vi "Autonomous Independent.vi"() -> ()   [LabVIEW 2015]
doc: "This VI is called when autonomous begins, and will automatically be terminated when autonomous ends. You can carry out timed or sensor driven robot movement independently without needing to return to the caller."
uses:
  <vilib>/Rock Robotics/WPI/Solenoid/WPI_SolenoidValue.ctl
  <vilib>/Rock Robotics/WPI/Relay/WPI_RelayValue.ctl
  <vilib>/Rock Robotics/WPI/Utilities/WPI_GetSetVariantRefNum.vi
  <vilib>/Rock Robotics/Network Tables/NT Read String.vi
  <vilib>/Rock Robotics/WPI/RobotDrive/WPI_RobotDriveArcadeDrive_Standard(NoSaturation).vi
  <vilib>/Rock Robotics/Network Tables/NT Write Numeric Array.vi
  <vilib>/Rock Robotics/WPI/Solenoid/WPI_SolenoidSetEnum.vi
  Robot Global Data.vi
panel:
  out "Current Movement, for debugging":T1 {"Y Joystick Value" scale=1.0..-1.0; "X Joystick Value" scale=-1.0..1.0}
  in  "Array of robot movements":T2(array[cluster])=[{"X Joystick Value"=0.39393939393939403, "Y Joystick Value"=0.0, "Delay (sec)"=1.0, "Movement Name"="turn"}, {"X Joystick Value"=-0.3737373737373737, "Y Joystick Value"=0.0, "Delay (sec)"=1.0, "Movement Name"="turn back"}] {"Y Joystick Value" scale=1.0..-1.0; "X Joystick Value" scale=-1.0..1.0}
  # "Be sure to right-click and choose Data Operations>>Make Current Value default if you want to save the array values with the VI"
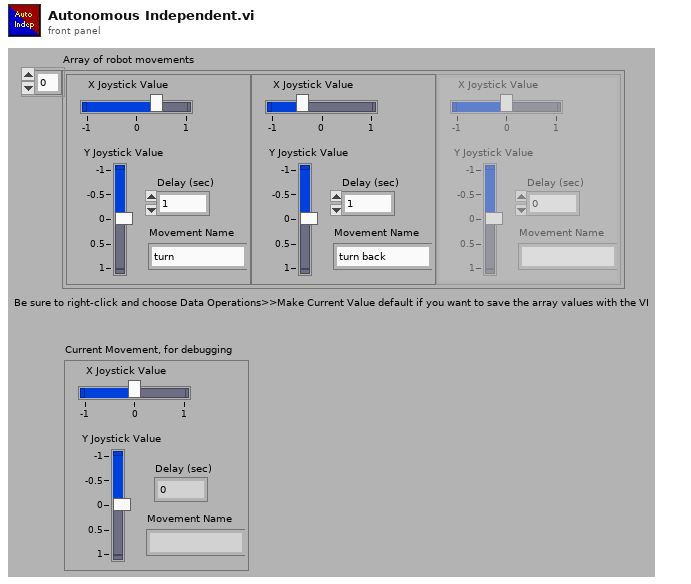
[diagram p1: front panel]
types:
  T1 = cluster{"X Joystick Value":dbl, "Y Joystick Value":dbl, "Delay (sec)":dbl, "Movement Name":string}
  T2 = cluster{"X Joystick Value":dbl, "Y Joystick Value":dbl, "Delay (sec)":dbl, "Movement Name":string}[]
  T3 = typedef "WPI_JoystickDevRef.ctl" = cluster{"Device":T4}
  T4 = typedef "WPI_JoystickDeviceEnum.ctl" = enum16{"USB 0", "USB 1", "USB 2", "USB 3", "USB 4", "USB 5"}
  T5 = typedef "WPI_RelayValue.ctl" = enum16{"Off", "On", "Forward", "Reverse"}
  T6 = typedef "WPI_SolenoidValue.ctl" = enum16{"Off", "On", "Forward", "Reverse"}
  T7 = typedef "WPI_RobotDriveDevRef.ctl" = cluster{"DevStatus":errorcluster, "Motors[]":T8[], "Square Inputs":bool, "Max Output":dbl}
  T8 = typedef "WPI_MotorControlDeviceRef.ctl" = cluster{"DeviceStatus":errorcluster, "Type":T9, "PWM":cluster{"PWM Channel":T10, "DeadBand":T11}, "CAN":cluster{"Device Number":u8, "Control Mode":T12, "Semaphore":T13, "Max Vout":dbl, "TalonSRX Control Mode":T14}, "Invert":bool}
  T9 = typedef "WPI_MotorControlType.ctl" = enum16{"PWM", "CAN", "CANTalonSRX"}
  T10 = typedef "FPGA_DIOPWMChannel.ctl" = enum8{"PWM 0", "PWM 1", "PWM 2", "PWM 3", "PWM 4", "PWM 5", "PWM 6", "PWM 7", "PWM 8", "PWM 9", "PWM MXP 0", "PWM MXP 1", "PWM MXP 2", "PWM MXP 3", "PWM MXP 4", "PWM MXP 5", "PWM MXP 6", "PWM MXP 7", "PWM MXP 8", "PWM MXP 9", "Invalid"}
  T11 = typedef "WPI_PWMDeadband.ctl" = cluster{"Name":string, "maxPositivePwm":i32, "minPositivePwm":i32, "centerPwm":i32, "maxNegativePwm":i32, "minNegativePwm":i32, "angularRange":u16}
  T12 = typedef "WPI_CANJaguar_ControlMode.ctl" = enum8{"Percent VBus", "Current", "Speed", "Position", "Voltage"}
  T13 = typedef "Semaphore RefNum" = refnum<k1>
  T14 = typedef "WPI_CANTalonSRX_APIControlMode.ctl" = enum8{"Percent VBus", "Speed", "Position", "Slave", "Unchanged / Invalid", "Voltage Compensation", "Current", "Motion Profile"}
  T15 = typedef "WPI_RelayDevRef.ctl" = cluster{"DevStatus":errorcluster, "Relay Channel":T16, "Relay Direction":T17}
  T16 = typedef "FPGA_DIORelayChannel.ctl" = enum8{"Relay 0", "Relay 1", "Relay 2", "Relay 3", "Invalid"}
  T17 = typedef "WPI_RelayDirection.ctl" = enum16{"Both directions", "Forward only", "Reverse only"}
  T18 = typedef "WPI_SolenoidDevRef.ctl" = cluster{"DevStatus":errorcluster, "Pneumatics Control Module":u8, "Forward Solenoid Channel":T19, "Reverse Solenoid Channel":T19}
  T19 = typedef "WPI_SolenoidChannel.ctl" = enum8{"Solenoid 0", "Solenoid 1", "Solenoid 2", "Solenoid 3", "Solenoid 4", "Solenoid 5", "Solenoid 6", "Solenoid 7", "Invalid"}
  T20 = cluster{"Distance (ft)":dbl, "Center":cluster{dbl, dbl}, "Normalized Rect":cluster{"Numeric":dbl, "Numeric 2":dbl, "Numeric 3":dbl, "Numeric 5":dbl}}[]
  T21 = cluster{"Distance (ft)":dbl, "Center":cluster{dbl, dbl}, "Normalized Rect":cluster{"Numeric":dbl, "Numeric 2":dbl, "Numeric 3":dbl, "Numeric 5":dbl}}
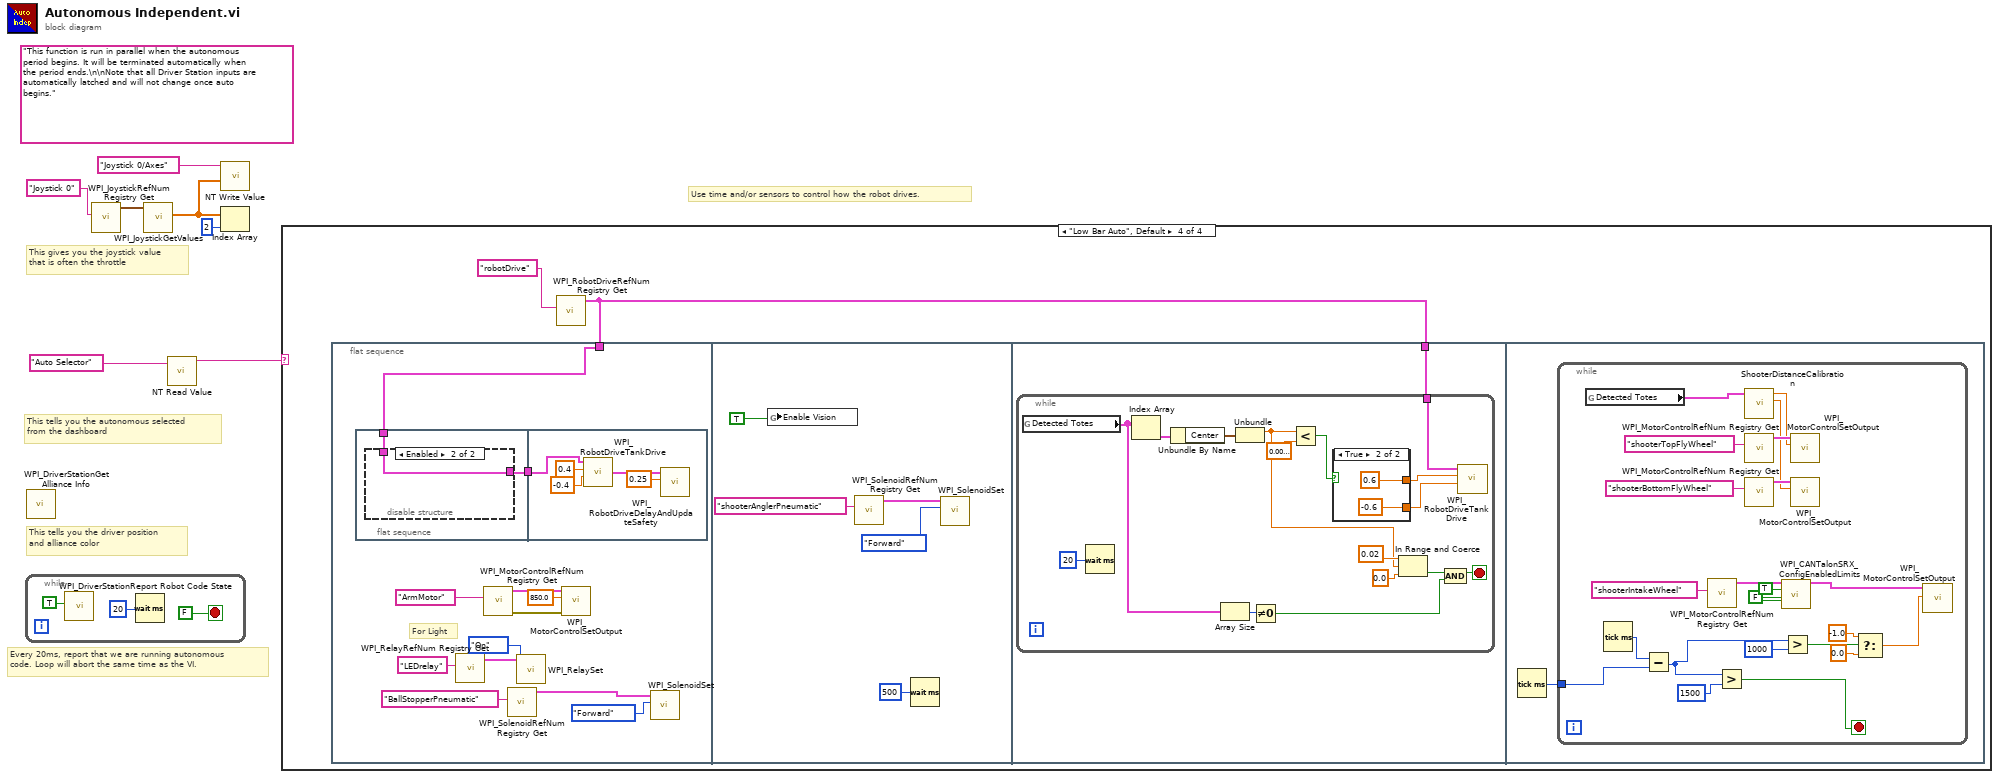
[diagram p0: block diagram]
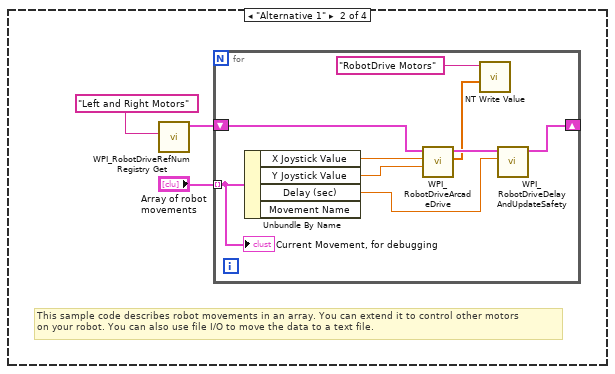
[diagram p3: hidden frame]
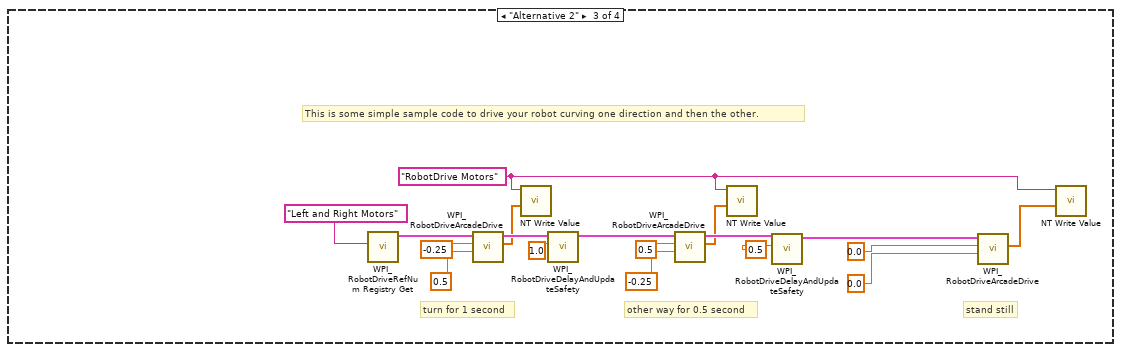
[diagram p4: hidden frame]
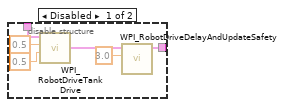
[diagram p5: hidden frame]
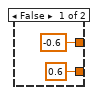
[diagram p6: hidden frame]
diagram:
  (unwired) "This function is run in parallel when the autonomous period begins. It will be terminated automatically when the period ends.\n\nNote that all Driver Station inputs are automatically latched and will not change once auto begins."
  # "This tells you the autonomous selected\nfrom the dashboard"
  # "Every 20ms, report that we are running autonomous\ncode. Loop will abort the same time as the VI."
  # "This gives you the joystick value\nthat is often the throttle"
  # "Use time and/or sensors to control how the robot drives."
  # "This tells you the driver position\nand alliance color"
  n1 = while {
    stop <- FALSE stop-if-true
    n2 = call <vilib>:"WPI_DriverStationReport Robot Code State.vi"("Autonomous"=TRUE) -> ()  [unwired: 10 in, 1 out]
    n3 = Wait (ms)(milliseconds to wait=u32 20) -> ()  [unwired: 1 out]
  }
  n4 = call <vilib>:"WPI_DriverStationGet Alliance Info.vi"() -> ()  [unwired: 12 out]
  n5 = call <vilib>:"WPI_JoystickRefNum Registry Get.vi"("refnum name"="Joystick 0") -> ("JoystickDevRef"=w6:T3)  [unwired: 1 in, 9 out]
  n6 = call <vilib>:"WPI_JoystickGetValues.vi"("JoystickDevRef"=w6) -> ("Axes"=w3:dbl[])  [unwired: 6 in, 4 out]
  n7 = call-poly <vilib>:"NT Read Value.vi"("Name"="Auto Selector") -> ("String"=w1:string)  [unwired: 9 in, 1 out]
  n8 = call-poly <vilib>:"NT Write Value.vi"("Numeric Array"=w3, "Name"="Joystick 0/Axes") -> ()  [unwired: 9 in, 1 out]
  n9 = Index Array(array=w3, index=2) -> ()  [unwired: 1 out]
  n10 = case shown="\"Low Bar Auto\", Default" w1 {
    frame "Nothing" {
      # "You can put your main auto here, or you can right-click on the case and make any\nother frame be the default case."
      # "This is the frame that will execute if no selection is made, or if it is not recognized"
    }
    frame "Alternative 1" {
      # "This sample code describes robot movements in an array. You can extend it to control other motors\non your robot. You can also use file I/O to move the data to a text file."
      n11 = call <vilib>:"WPI_RobotDriveRefNum Registry Get.vi"("refnum name"="Left and Right Motors") -> ("RobotDriveDevRef"=w12:T7)  [unwired: 1 in, 9 out]
      n12 = for {
        shift-right: [w20] -> _
        shift-left: w12 -> [w21]
        tunnel: "Array of robot movements" -> [w16] mode=indexing
        n13 = Unbundle By Name(w16) -> ("X Joystick Value"=w19:dbl, "Y Joystick Value"=w18:dbl, "Delay (sec)"=w17:dbl)  [unwired: 1 out]
        n14 = call-poly <vilib>:"WPI_RobotDriveArcadeDrive.vi"("Y axis value"=w18, "X axis value"=w19, "RobotDriveDevRef"=w21) -> ("Motor Values"=w14:dbl[], "RobotDriveDevRef"=w22:T7)  [unwired: 1 in, 6 out]
        n15 = call-poly <vilib>:"NT Write Value.vi"("Numeric Array"=w14, "Name"="RobotDrive Motors") -> ()  [unwired: 9 in, 1 out]
        n16 = call <vilib>:"WPI_RobotDriveDelayAndUpdateSafety.vi"("Delay (s)"=w17, "RobotDriveDevRef"=w22) -> ("RobotDriveDevRef 2"=w20:T7)  [unwired: 8 in, 1 out]
        "Current Movement, for debugging" <- w16
      }
    }
    frame "Alternative 2" {
      w24 = "RobotDrive Motors" ("Name")
      # "This is some simple sample code to drive your robot curving one direction and then the other."
      # "stand still"
      # "other way for 0.5 second"
      # "turn for 1 second"
      n17 = call <vilib>:"WPI_RobotDriveRefNum Registry Get.vi"("refnum name"="Left and Right Motors") -> ("RobotDriveDevRef"=w40:T7)  [unwired: 1 in, 9 out]
      n18 = call-poly <vilib>:"WPI_RobotDriveArcadeDrive.vi"("Y axis value"=0.5 ("X axis value"), "X axis value"=-0.25, "RobotDriveDevRef"=w40) -> ("Motor Values"=w23:dbl[], "RobotDriveDevRef"=w33:T7)  [unwired: 1 in, 6 out]
      n19 = call-poly <vilib>:"NT Write Value.vi"("Numeric Array"=w23, "Name"=w24) -> ()  [unwired: 9 in, 1 out]
      n20 = call <vilib>:"WPI_RobotDriveDelayAndUpdateSafety.vi"("Delay (s)"=1.0, "RobotDriveDevRef"=w33) -> ("RobotDriveDevRef 2"=w34:T7)  [unwired: 8 in, 1 out]
      n21 = call-poly <vilib>:"WPI_RobotDriveArcadeDrive.vi"("Y axis value"=-0.25 ("X axis value"), "X axis value"=0.5, "RobotDriveDevRef"=w34) -> ("Motor Values"=w25:dbl[], "RobotDriveDevRef"=w35:T7)  [unwired: 1 in, 6 out]
      n22 = call-poly <vilib>:"NT Write Value.vi"("Numeric Array"=w25, "Name"=w24) -> ()  [unwired: 9 in, 1 out]
      n23 = call <vilib>:"WPI_RobotDriveDelayAndUpdateSafety.vi"("Delay (s)"=0.5, "RobotDriveDevRef"=w35) -> ("RobotDriveDevRef 2"=w36:T7)  [unwired: 8 in, 1 out]
      n24 = call-poly <vilib>:"WPI_RobotDriveArcadeDrive.vi"("Y axis value"=0.0 ("X axis value"), "X axis value"=0.0, "RobotDriveDevRef"=w36) -> ("Motor Values"=w26:dbl[])  [unwired: 1 in, 7 out]
      n25 = call-poly <vilib>:"NT Write Value.vi"("Numeric Array"=w26, "Name"=w24) -> ()  [unwired: 9 in, 1 out]
    }
    frame "Low Bar Auto", Default {
      n26 = flat-sequence {
        tunnel: w41 -> [w54]
        tunnel: w41 -> [w74]
        frame #0 {
          # "For Light"
          n27 = flat-sequence {
            tunnel: w54 -> [w56]
            tunnel: [w55] -> w50
            tunnel: w50 -> [w64]
            frame #0 {
              n28 = disable-structure shown="Enabled" {
                disable-tunnel: w56 -> [w58 w63]
                disable-tunnel: [w57 w63] -> w55
                frame Disabled {
                  n29 = call <vilib>:"WPI_RobotDriveTankDrive.vi"("Right axis value"=0.5, "Left axis value"=0.5, "RobotDriveDevRef"=w58) -> ("RobotDriveDevRef"=w61:T7)  [unwired: 6 in, 2 out]
                  n30 = call <vilib>:"WPI_RobotDriveDelayAndUpdateSafety.vi"("Delay (s)"=3.0, "RobotDriveDevRef"=w61) -> ("RobotDriveDevRef 2"=w57:T7)  [unwired: 8 in, 1 out]
                }
                frame Enabled {
                }
              }
            }
            frame #1 {
              n31 = call <vilib>:"WPI_RobotDriveTankDrive.vi"("Right axis value"=-0.4, "Left axis value"=0.4, "RobotDriveDevRef"=w64) -> ("RobotDriveDevRef"=w67:T7)  [unwired: 6 in, 2 out]
              n32 = call <vilib>:"WPI_RobotDriveDelayAndUpdateSafety.vi"("Delay (s)"=0.25, "RobotDriveDevRef"=w67) -> ()  [unwired: 8 in, 2 out]
            }
          }
          n33 = call <vilib>:"WPI_RelayRefNum Registry Get.vi"("refnum name"="LEDrelay") -> ("RelayDevRef"=w44:T15)  [unwired: 9 in, 1 out]
          n34 = call <vilib>:"WPI_MotorControlRefNum Registry Get.vi"("refnum name"="ArmMotor") -> ("error out"=w49:errorcluster, "MotorControlDevRef"=w47:T8)  [unwired: 9 in]
          n35 = call <vilib>:"WPI_SolenoidRefNum Registry Get.vi"("refnum name"="BallStopperPneumatic") -> ("SolenoidDevRef"=w51:T18)  [unwired: 9 in, 1 out]
          n36 = call <vilib>:"WPI_RelaySet.vi"("RelayValue"=WPI_RelayValue."On", "RelayDevRef"=w44) -> ()  [unwired: 8 in, 2 out]
          n37 = call <vilib>:"WPI_MotorControlSetOutput.vi"("error in (no error)"=w49, "Output"=850.0, "MotorControlDevRef"=w47) -> ()  [unwired: 6 in, 3 out]
          n38 = call-poly <vilib>:"WPI_SolenoidSet.vi"("Value"=WPI_SolenoidValue."Forward", "SolenoidDevRef"=w51) -> ()  [unwired: 8 in, 2 out]
        }
        frame #1 {
          n39 = global write "Robot Global Data.vi" "Enable Vision"(TRUE ("Enable Vision")) -> ()
          n40 = call <vilib>:"WPI_SolenoidRefNum Registry Get.vi"("refnum name"="shooterAnglerPneumatic") -> ("SolenoidDevRef"=w71:T18)  [unwired: 9 in, 1 out]
          n41 = Wait (ms)(milliseconds to wait=u32 500) -> ()  [unwired: 1 out]
          n42 = call-poly <vilib>:"WPI_SolenoidSet.vi"("Value"=WPI_SolenoidValue."Forward", "SolenoidDevRef"=w71) -> ()  [unwired: 8 in, 2 out]
        }
        frame #2 {
          n43 = while {
            tunnel: w74 -> [w85]
            stop <- w81 stop-if-true
            n44 = global read "Robot Global Data.vi" "Detected Totes"() -> (w80:T20)
            n45 = Wait (ms)(milliseconds to wait=u32 20) -> ()  [unwired: 1 out]
            n46 = Index Array(array=w80) -> (element=w90:T21)  [unwired: 1 in]
            n47 = Unbundle By Name(w90) -> ("Center"=w89:cluster{dbl, dbl})
            n48 = Array Size(array=w80) -> (size(s)=w79:i32)
            n49 = Unbundle(w89) -> (w76:dbl)  [unwired: 1 out]
            n50 = Not Equal To 0?(x=w79) -> (x != 0?=w78:bool)
            n51 = Less?(x=w76, y=0.009999999999999997 ("x")) -> (x < y?=w84:bool)
            n52 = case shown="True" w84 {
              tunnel: [0.6 ("Left axis value") -0.6 ("Left axis value")] -> w83
              tunnel: [-0.6 ("Left axis value") 0.6 ("Left axis value")] -> w82
              frame False {
              }
              frame True {
              }
            }
            n53 = In Range and Coerce(upper limit=0.02, x=w76, lower limit=0.0) -> (In Range?=w86:bool)  [unwired: 1 out]
            n54 = Compound Arithmetic op=AND(w86, w78) -> (w81:bool)
            n55 = call <vilib>:"WPI_RobotDriveTankDrive.vi"("Right axis value"=w83, "Left axis value"=w82, "RobotDriveDevRef"=w85) -> ()  [unwired: 6 in, 3 out]
          }
        }
        frame #3 {
          n56 = Tick Count (ms)() -> (millisecond timer value=w95:u32)
          n57 = while {
            tunnel: w95 -> [w115]
            stop <- w113 stop-if-true
            w96 = FALSE ("Forward Limit Switch Enable")
            n58 = global read "Robot Global Data.vi" "Detected Totes"() -> (w108:T20)
            n59 = Tick Count (ms)() -> (millisecond timer value=w116:u32)
            n60 = Subtract(x=w116, y=w115) -> (x-y=w107:u32)
            n61 = call <vilib>:"WPI_MotorControlRefNum Registry Get.vi"("refnum name"="shooterIntakeWheel") -> ("MotorControlDevRef"=w99:T8)  [unwired: 9 in, 1 out]
            n62 = Greater?(x=w107, y=u32 1500) -> (0:w113:bool)
            n63 = call "ShooterDistanceCalibration.vi"("Detected Totes"=w108) -> ("bottomFlyWheelConstant"=w109:dbl, "TopFlyWheelConstant"=w110:dbl)  [unwired: 9 in]
            n64 = call <vilib>:"WPI_MotorControlRefNum Registry Get.vi"("refnum name"="shooterTopFlyWheel") -> ("MotorControlDevRef"=w111:T8)  [unwired: 9 in, 1 out]
            n65 = call <vilib>:"WPI_MotorControlRefNum Registry Get.vi"("refnum name"="shooterBottomFlyWheel") -> ("MotorControlDevRef"=w112:T8)  [unwired: 9 in, 1 out]
            n66 = call <vilib>:"WPI_CANTalonSRX_ConfigEnabledLimits.vi"("CAN Talon SRX Ref"=w99, "Override Limit Switches"=TRUE, "Forward Limit Switch Enable"=w96, "Reverse Limit Switch Enable"=w96) -> ("CAN Talon SRX Ref"=w98:T8)  [unwired: 10 in, 1 out]
            n67 = Greater?(x=w107, y=u32 1000) -> (0:w105:bool)
            n68 = call <vilib>:"WPI_MotorControlSetOutput.vi"("Output"=w110, "MotorControlDevRef"=w111) -> ()  [unwired: 7 in, 3 out]
            n69 = call <vilib>:"WPI_MotorControlSetOutput.vi"("Output"=w109, "MotorControlDevRef"=w112) -> ()  [unwired: 7 in, 3 out]
            n70 = Select(t=-1.0, s=w105, f=0.0) -> (s? t:f=w102:dbl)
            n71 = call <vilib>:"WPI_MotorControlSetOutput.vi"("Output"=w102, "MotorControlDevRef"=w98) -> ()  [unwired: 7 in, 3 out]
          }
        }
      }
      n72 = call <vilib>:"WPI_RobotDriveRefNum Registry Get.vi"("refnum name"="robotDrive") -> ("RobotDriveDevRef"=w41:T7)  [unwired: 9 in, 1 out]
    }
  }
